vi "select vi.vi"(1 "Beamline Section":T1, 2 "error in (no error)":errorcluster, 3 "reference":refnum<vi>) -> (0 "error out":errorcluster)   [LabVIEW 2016, in "main.lvlib"]
doc: "Selects which vi is displayed in the sub panel"
uses:
  main.lvlib
  beamline selection.ctl
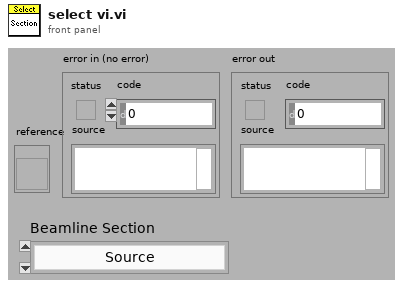
[diagram p1: front panel]
types:
  T1 = typedef "main.lvlib/beamline selection.ctl" = enum16{"Source", "Low End", "High End", "Transmission", "R30", "R45"}
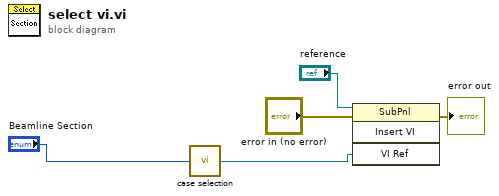
[diagram p0: block diagram]
diagram:
  n1 = call "case selection.vi"("Beamline Section"="Beamline Section") -> ("VI Refnum"=w5:refnum<vi>)
  n2 = invoke on="Invoke Node" class="SubPnl" method="Insert VI"(reference="reference", error in="error in (no error)", "VI Ref"=w5) -> (error out=→"error out":errorcluster)  [unwired: 1 in, 3 out]
